vi "error_handler.vi"(8 "error in (no error)":errorcluster) -> ()   [LabVIEW 2017]
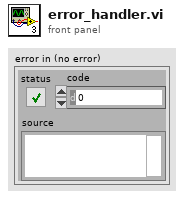
[diagram p1: front panel]
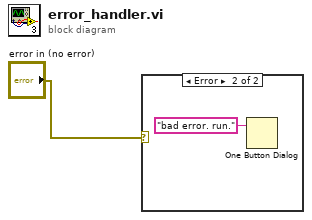
[diagram p0: block diagram]
diagram:
  n1 = case shown="Error" "error in (no error)" {
    frame No Error {
    }
    frame Error {
      n2 = One Button Dialog(message="bad error. run.") -> ()  [unwired: 1 in, 1 out]
    }
  }
